vi "Window-Parameters entry dialogue.vi"(9 "AVI playback header info cluster":T1, 11 "Message":string="This dataset's header file could not be loaded.\nPlease enter the following information about this dataset for the playback to work at the correct speed.") -> (0 "error out":errorcluster, 1 "Cancelled":bool)   [LabVIEW 2017]
doc: "Use this template to create a dialog box with event handling."
uses:
  Typedefs/Frame Size.ctl
  Typedefs/AVI playback header info cluster.ctl
  <vilib>/Utility/miscctls.llb/LVPointTypeDef.ctl
  Globals/gl_Time series viewer globals.vi
  Global Variables/General Globals.vi
panel:
  in  "Frame Size":T2=512 items=["100X100"=100, "128X128"=128, "200X200"=200, "256X256"=256, "512X512"=512, "1024x1024"=1024, "2048x2048"=2048]
  in  "Dwell time (us)":dbl=0.05 min=0.01 max=100.0 step=0.05
  in  "AOD fill time (us)":dbl=1.0 min=1.0 max=100.0 step=0.5
  in  "Cancel":bool
  in  "OK":bool
  out "Message ind":string="This dataset's header file could not be loaded.\nPlease enter the following information about this dataset for the playback to work at the correct/original speed."
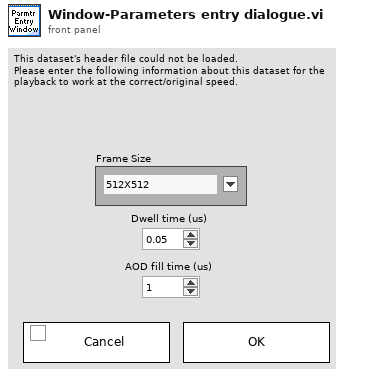
[diagram p1: front panel]
types:
  T1 = typedef "AVI playback header info cluster.ctl" = cluster{"Frame Size":u32, "AOD fill time (us)":dbl, "Dwell time (us)":dbl, "Frame period (ms)":dbl, "Number of Miniscans":u16, "Number of Pixels in Miniscan":u16}
  T2 = typedef "Frame Size.ctl" = u16
  T3 = typedef "LVPointTypeDef.ctl" = cluster{"Horizontal":i16, "Vertical":i16}
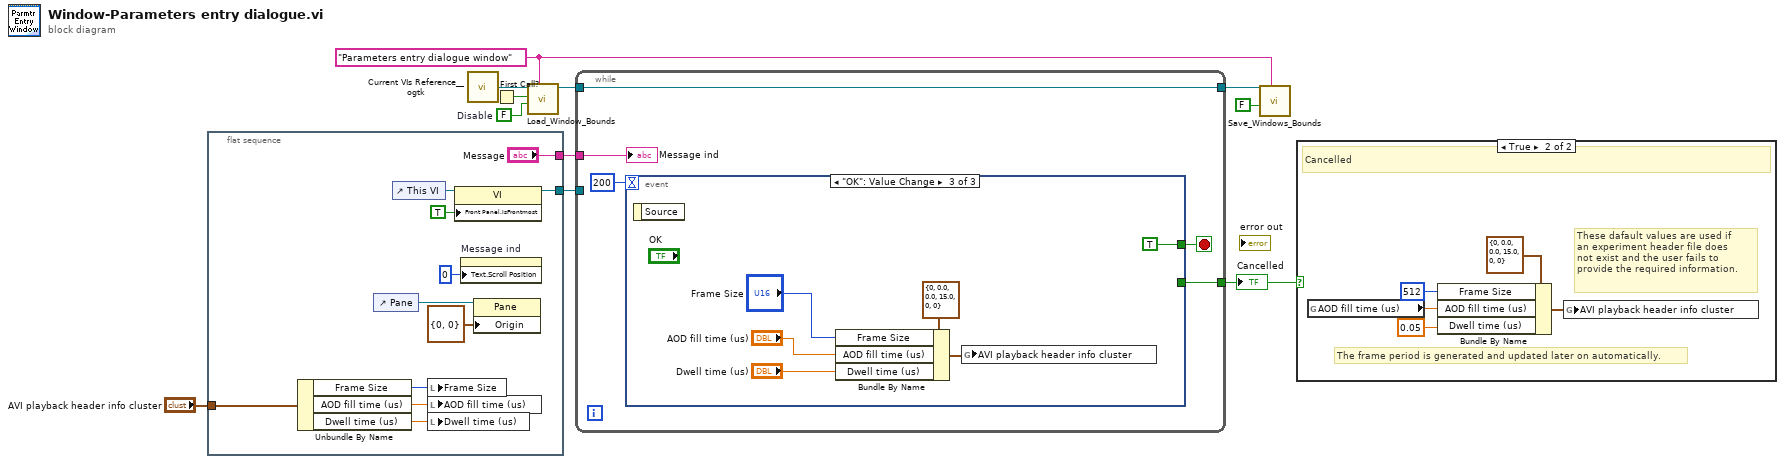
[diagram p0: block diagram]
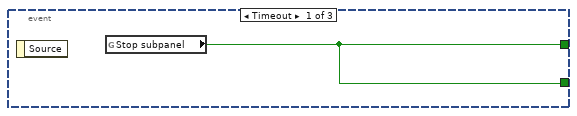
[diagram p3: hidden frame]
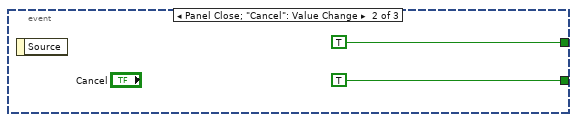
[diagram p4: hidden frame]
diagram:
  w5 = FALSE  # Disable
  w4 = "Parameters entry dialogue window" ("Window Name (i.e. Key)")
  n1 = flat-sequence {
    tunnel: [w19] -> w11
    tunnel: ["Message"] -> w9
    tunnel: "AVI playback header info cluster" -> [w15]
    frame #0 {
      n2 = Unbundle By Name(w15) -> ("Frame Size"=w14:u32, "AOD fill time (us)"=w13:dbl, "Dwell time (us)"=w12:dbl)
      n3 = control-ref of="Pane"() -> (w17:refnum<vi>)
      n4 = control-ref of="This VI"() -> (w20:refnum<vi>)
      n5 = local write "Frame Size"(w14) -> ()
      n6 = local write "AOD fill time (us)"(w13) -> ()
      n7 = local write "Dwell time (us)"(w12) -> ()
      n8 = property on="Property Node" class="VI"(reference=w20, "Front Panel.IsFrontmost"=TRUE ("Front Panel Window:Is Frontmost")) -> (reference out=w19:refnum<vi>)  [unwired: 1 in, 1 out]
      n9 = property on="Message ind" class="Str"("Text.Scroll Position"=u32 0) -> ()  [unwired: 2 in, 2 out]
      n10 = property class="Pane"(reference=w17, "Origin"=T3 {"Horizontal"=0, "Vertical"=0}) -> ()  [unwired: 1 in, 2 out]
    }
  }
  n11 = call <userlib>:"Current VIs Reference__ogtk.vi"() -> ("Current VI's reference"=w7:refnum<vi>)  [unwired: 5 in]
  n12 = First Call?() -> (First Call?: T/F=w6:bool)
  n13 = call "Load_Window_Bounds.vi"("Window Name (i.e. Key)"=w4, "Disable"=w5, "First Call"=w6, "Window VI's Ref"=w7) -> ("reference out"=w2:refnum<vi>)  [unwired: 4 in, 3 out]
  n14 = while {
    tunnel: w11 -> [_]
    tunnel: [w25] -> w10
    tunnel: w9 -> [w24]
    tunnel: w2 -> [w23]
    tunnel: [w23] -> w1
    stop <- w27 stop-if-true
    n15 = event shown="[2] \"OK\": Value Change" {
      selector: _ -> [_ _ _]
      dyn-events: _ -> [_ _ _]
      timeout: 200 -> [_ _ _]
      tunnel: [w28 TRUE ("Stop?") TRUE ("Stop?")] -> w27
      tunnel: [w28 TRUE ("Stop subpanel") _] -> w25
      event Timeout {
        n16 = event-data() -> ()  [unwired: 1 in, 1 out]
        n17 = global read "General Globals.vi" "Stop subpanel"() -> (w28:bool)
      }
      event Panel Close; "Cancel": Value Change {
        n18 = event-data() -> ()  [unwired: 1 in, 1 out]
      }
      event "OK": Value Change {
        n19 = event-data() -> ()  [unwired: 1 in, 1 out]
        n20 = Bundle By Name(cluster=T1 {"Frame Size"=0, "AOD fill time (us)"=0.0, "Dwell time (us)"=0.0, "Frame period (ms)"=15.0, "Number of Miniscans"=0, "Number of Pixels in Miniscan"=0} ("AVI playback header info cluster"), "Frame Size"="Frame Size", "AOD fill time (us)"="AOD fill time (us)", "Dwell time (us)"="Dwell time (us)") -> (w31:T1)
        n21 = global write "gl_Time series viewer globals.vi" "AVI playback header info cluster"(w31) -> ()
      }
    }
    "Message ind" <- w24
  }
  "Cancelled" <- w10
  n22 = call "Save_Windows_Bounds.vi"("Window Name (i.e. Key)"=w4, "Front Panel Window:Open"=FALSE, "Window VI's Ref"=w1) -> ()  [unwired: 8 in, 1 out]
  n23 = case shown="True" w10 {
    frame False {
    }
    frame True {
      # "The frame period is generated and updated later on automatically."
      # "These dafault values are used if \nan experiment header file does \nnot exist and the user fails to provide the required information."
      # "Cancelled"
      n24 = global read "General Globals.vi" "AOD fill time (us)"() -> (w38:dbl)
      n25 = Bundle By Name(cluster=T1 {"Frame Size"=0, "AOD fill time (us)"=0.0, "Dwell time (us)"=0.0, "Frame period (ms)"=15.0, "Number of Miniscans"=0, "Number of Pixels in Miniscan"=0} ("AVI playback header info cluster"), "Frame Size"=u32 512, "AOD fill time (us)"=w38, "Dwell time (us)"=0.05) -> (w41:T1)
      n26 = global write "gl_Time series viewer globals.vi" "AVI playback header info cluster"(w41) -> ()
    }
  }
